vi "Coord window-Shortcut menu activation handler.vi"(9 "MenuRef":refnum<k9>, 10 "Coords":T1, 11 "MulticolumnListbox in":refnum<vi>) -> (0 "error out":errorcluster, 1 "Menu out":refnum<k9>, 2 "Clicked on empty row":bool, 3 "MulticolumnListbox out":refnum<vi>)   [LabVIEW 2017]
uses:
  <vilib>/Utility/miscctls.llb/LVPoint32TypeDef.ctl
  Globals/Coord window-Globals.vi
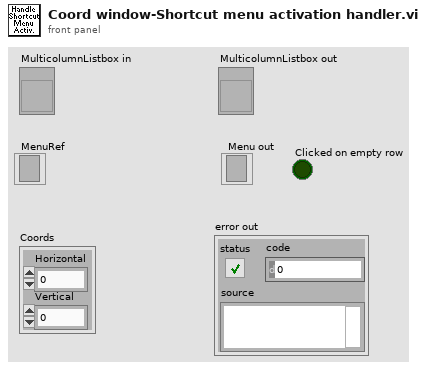
[diagram p1: front panel]
types:
  T1 = typedef "LVPoint32TypeDef.ctl" = cluster{"Horizontal":i32, "Vertical":i32}
  T2 = typedef "LVRowAndColumnTypeDef.ctl" = cluster{"Row":i32, "Column":i32}
  T3 = typedef "Test_Header_Info_MC_Listbox.ctl" = i32[]
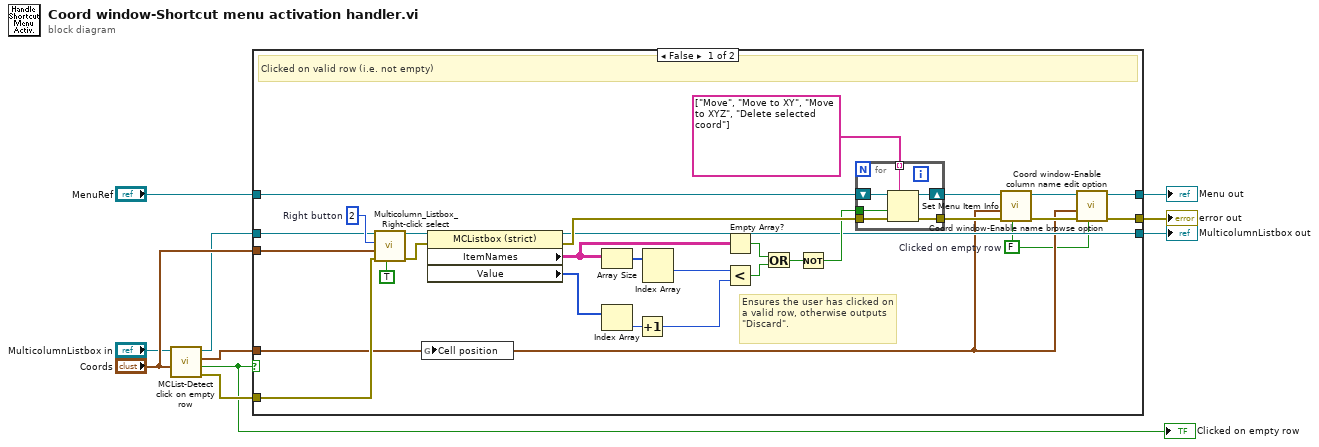
[diagram p0: block diagram]
diagram:
  n1 = call "MCList-Detect click on empty row.vi"("Coords"="Coords", "MulticolumnListbox in"="MulticolumnListbox in") -> ("error out"=w2:errorcluster, "Clicked on empty row"=w1:bool, "Cell Position"=w6:T2, "MulticolumnListbox out"=w5:refnum<vi>)  [unwired: 6 in]
  "Clicked on empty row" <- w1
  n2 = case shown="False" w1 {
    tunnel: "MenuRef" -> [w13 w48]
    tunnel: [w16 w47] -> w9
    tunnel: [w17 w48] -> w8
    tunnel: "Coords" -> [w26 _]
    tunnel: w6 -> [w15 _]
    tunnel: w5 -> [w24 w46]
    tunnel: [w23 w46] -> w3
    tunnel: w2 -> [w22 w47]
    frame False {
      w14 = FALSE  # Clicked on empty row
      w25 = u16 2  # Right button
      # "Ensures the user has clicked on a valid row, otherwise outputs \"Discard\"."
      # "Clicked on valid row (i.e. not empty)"
      n3 = call <userlib>:"Multicolumn_Listbox_Right-click select.vi"("Disable when multiple selection"=TRUE, "error in (no error)"=w22, "Coords"=w26, "Button"=w25, "MulticolumnListbox in"=w24) -> ("error out"=w29:errorcluster, "MulticolumnListbox out"=w36:refnum<vi>)  [unwired: 5 in]
      n4 = global write "Coord window-Globals.vi" "Cell position"(w15) -> ()
      n5 = property on="Property Node" class="MCListbox (strict)"(reference=w36, error in=w29) -> (reference out=w23:refnum<vi>, error out=w28:errorcluster, "ItemNames"=w35:string[][], "Value"=w21:T3)
      n6 = Array Size(array=w35) -> (size(s)=w37:i32[])
      n7 = Index Array(array=w21) -> (element=w38:i32)  [unwired: 1 in]
      n8 = Increment(x=w38) -> (x+1=w20:i32)
      n9 = Index Array(array=w37) -> (element #1=w39:i32)  [unwired: 2 in, 1 out]
      n10 = Empty Array?(array=w35) -> (empty?=w34:bool)
      n11 = Less?(x=w39, y=w20) -> (x < y?=w33:bool)
      n12 = Or(x=w34, y=w33) -> (x .or. y?=w32:bool)
      n13 = Not(x=w32) -> (.not. x?=w27:bool)
      n14 = for {
        tunnel: [w44] -> w30
        tunnel: w28 -> [w43]
        tunnel: w27 -> [w42]
        shift-right: [w45] -> w31
        shift-left: w13 -> [w41]
        tunnel: string[] ["Move", "Move to XY", "Move to XYZ", "Delete selected coord"] -> [w40] mode=indexing
        n15 = Set Menu Item Info(7:w40, 8:w43, 9:w42, 11:w41) -> (0:w44:errorcluster, 3:w45:refnum<k9>)  [unwired: 3 in]
      }
      n16 = call "Coord window-Enable name browse option.vi"("Clicked on empty row"=w14, "error in (no error)"=w30, "Cell Position"=w15, "Menu in"=w31) -> ("error out"=w18:errorcluster, "Menu out"=w19:refnum<k9>)  [unwired: 6 in]
      n17 = call "Coord window-Enable column name edit option.vi"("Clicked on empty row"=w14, "error in (no error)"=w18, "Cell Position"=w15, "Menu in"=w19) -> ("error out"=w16:errorcluster, "Menu out"=w17:refnum<k9>)  [unwired: 6 in]
    }
    frame True {
      # "Clicked on empty row"
    }
  }
  "error out" <- w9
  "MulticolumnListbox out" <- w3
  "Menu out" <- w8
